vi "PMBus Set Control.vi"(7 "Value":u8, 9 "PMBusIndex":i32, 10 "DevIndex":i32, 11 "DevType":i32) -> (3 "function return":i32)   [LabVIEW 2010, in "ControlPMBus.lvlib"]
doc: "int WINAPI PMBus_SetControl(int DevType,int DevIndex,int PMBusIndex,unsigned char Value);"
uses:
  ControlPMBus.lvlib
  ControlPMBus/Ginkgo_Driver.dll
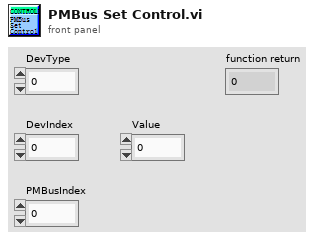
[diagram p1: front panel]
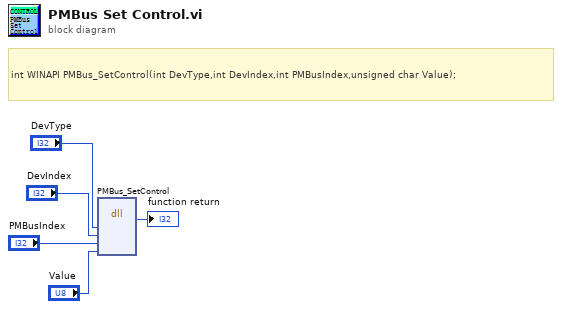
[diagram p0: block diagram]
diagram:
  # "int WINAPI PMBus_SetControl(int DevType,int DevIndex,int PMBusIndex,unsigned char Value);"
  n1 = dll-call lib="E:/Project/vt_ginkgo/truck/Ginkgo Driver/vs2010/Ginkgo_USB-I2C&SPI&CAN_API_v2.0.3.3/lib/labview_32bit/ControlPMBus/Ginkgo_Driver.*" fn="PMBus_SetControl"("DevType"="DevType", "DevIndex"="DevIndex", "PMBusIndex"="PMBusIndex", "Value"="Value") -> (→"function return":i32)  [unwired: 7 in, 2 out]
